vi "CRYTS Step Select.vi"(11 "Tree reference In":refnum<vi>) -> (0 "nData_Out":i32, 2 "sData_Out":string)   [LabVIEW 2013]
uses:
  CRYProject Editor Global.vi
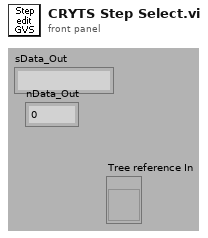
[diagram p1: front panel]
types:
  T1 = typedef "CRYTS.ctl" = cluster{"No.TS":u16, "TS File Path":path, "TS Name":string, "EditStepName":string, "Steps":T2[], "New State":bool, "Change State":bool, "Flattened CurveLib Data":string, "Document Data":string, "EditStepNo":u16, "Operator Start File":string, "Sequence Type":string, "Sequence Language":string}
  T2 = typedef "CRYStep.ctl" = cluster{"No.VI":i32, "Category":string, "StepName":string, "Seq setup flattened":string, "Comment":string, "Steps config.":bool[], "Jump config":i32[], "Start":dbl, "Increment":dbl, "Name":string, "Unit":string, "Y data":u16, "Y prefix":string, "Y dB ref":dbl, "Y unit":string, "Repeat State Array":cluster{"Start":dbl, "Increment":dbl, "Count":i32, "Num":i32}[]}
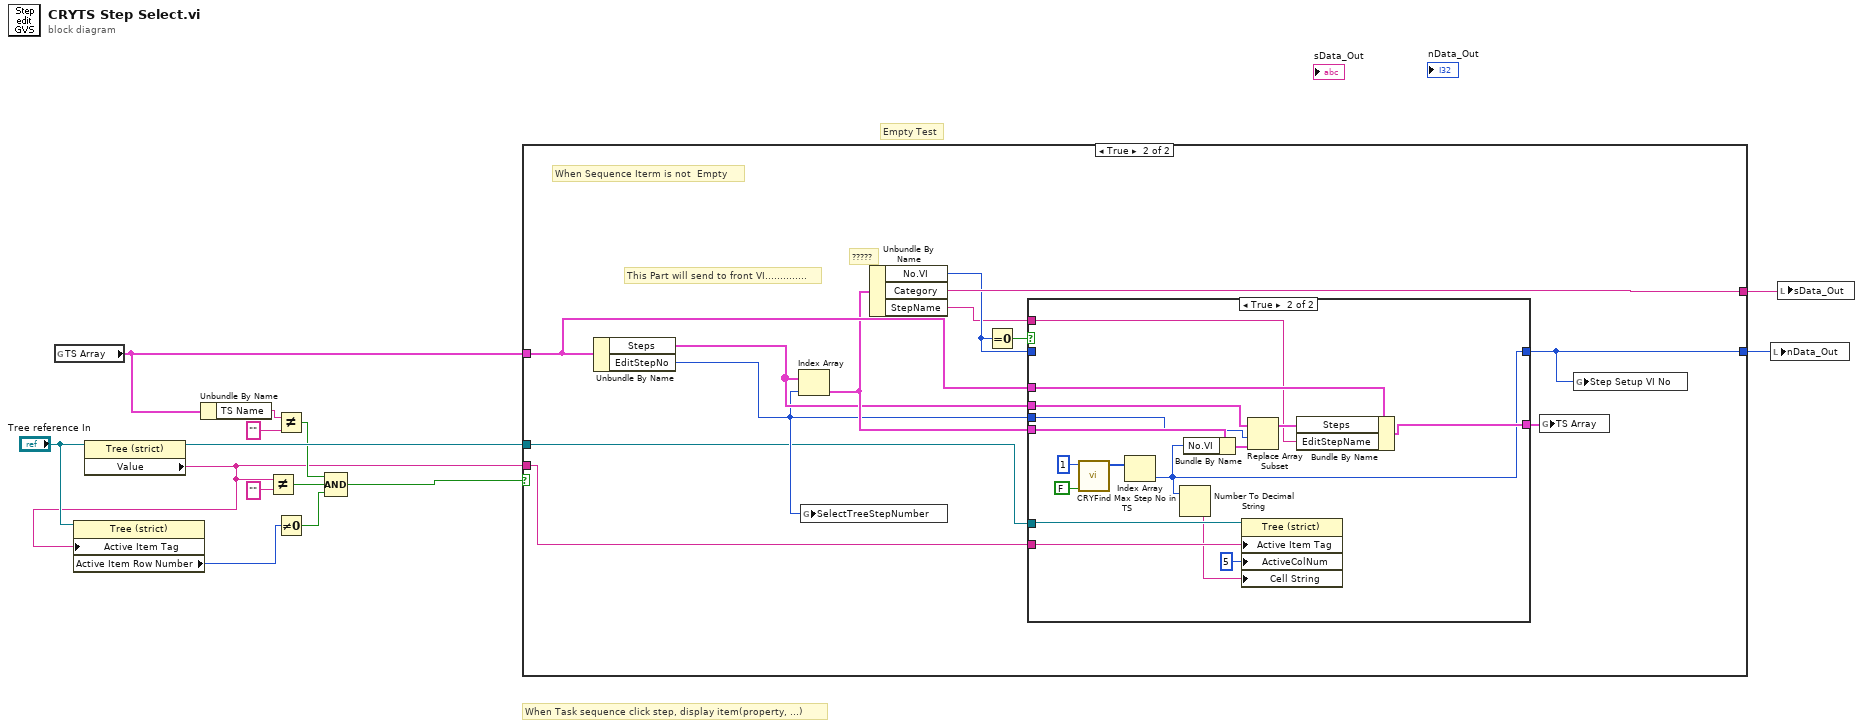
[diagram p0: block diagram]
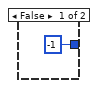
[diagram p2: hidden frame]
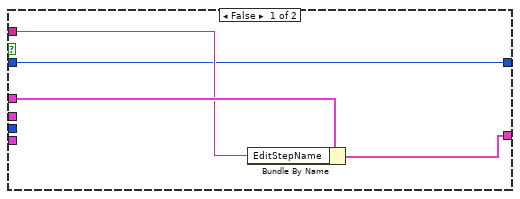
[diagram p3: hidden frame]
diagram:
  # "Empty Test"
  # "When Task sequence click step, display item(property, ...)"
  n1 = global read "CRYProject Editor Global.vi" "TS Array"() -> (w7:T1)
  n2 = property on="Property Node" class="Tree (strict)"(reference="Tree reference In") -> (reference out=w13:refnum<vi>, "Value"=w2:string)  [unwired: 1 in, 1 out]
  n3 = property on="Property Node" class="Tree (strict)"(reference="Tree reference In", "Active Item Tag"=w2) -> ("Active Item Row Number"=w1:i32)  [unwired: 1 in, 2 out]
  n4 = Unbundle By Name(w7) -> ("TS Name"=w12:string)
  n5 = Not Equal?(x=w2, y="") -> (x != y?=w10:bool)
  n6 = Not Equal?(x=w12, y="") -> (x != y?=w9:bool)
  n7 = Not Equal To 0?(x=w1) -> (x != 0?=w4:bool)
  n8 = Compound Arithmetic op=AND(w9, w10, w4) -> (w11:bool)
  n9 = case shown="True" w11 {
    tunnel: w2 -> [_ w16]
    tunnel: w13 -> [_ w17]
    tunnel: [_ w27] -> w6
    tunnel: w7 -> [_ w26]
    tunnel: [-1 ("Max Number") w25] -> w5
    frame False {
    }
    frame True {
      # "This Part will send to front VI.............."
      # "?????"
      # "When Sequence Iterm is not  Empty"
      n10 = Unbundle By Name(w26) -> ("Steps"=w19:T2[], "EditStepNo"=w18:u16)
      n11 = Index Array(array=w19, index=w18) -> (element=w23:T2)
      n12 = global write "CRYProject Editor Global.vi" "SelectTreeStepNumber"(w18) -> ()
      n13 = Unbundle By Name(w23) -> ("No.VI"=w22:i32, "Category"=w27:string, "StepName"=w21:string)
      n14 = Equal To 0?(x=w22) -> (x = 0?=w24:bool)
      n15 = case shown="True" w24 {
        tunnel: [w28 w34] -> w25
        tunnel: w22 -> [w28 _]
        tunnel: w18 -> [_ w37]
        tunnel: w23 -> [_ w47]
        tunnel: w19 -> [_ w45]
        tunnel: w26 -> [w31 w44]
        tunnel: w21 -> [w30 w42]
        tunnel: [w29 w41] -> w20
        tunnel: w17 -> [_ w36]
        tunnel: w16 -> [_ w35]
        frame False {
          n16 = Bundle By Name(cluster=w31, "EditStepName"=w30) -> (w29:T1)
        }
        frame True {
          n17 = call "CRYFind Max Step No in TS.vi"("Inputflg"=FALSE, "Required Count"=1) -> ("Num Array Out"=w39:i32[])  [unwired: 1 in, 8 out]
          n18 = Index Array(array=w39) -> (element=w34:i32)  [unwired: 1 in]
          n19 = Number To Decimal String(number=w34) -> (decimal integer string=w33:string)  [unwired: 1 in]
          n20 = Bundle By Name(cluster=w47, "No.VI"=w34) -> (w46:T2)
          n21 = property class="Tree (strict)"(reference=w36, "Active Item Tag"=w35, "ActiveColNum"=5 ("Active Cell:Active Column Number"), "Cell String"=w33) -> ()  [unwired: 1 in, 2 out]
          n22 = Replace Array Subset(array=w45, new element=w46, index=w37) -> (w43:T2[])
          n23 = Bundle By Name(cluster=w44, "Steps"=w43, "EditStepName"=w42) -> (w41:T1)
        }
      }
      n24 = global write "CRYProject Editor Global.vi" "TS Array"(w20) -> ()
      n25 = global write "CRYProject Editor Global.vi" "Step Setup VI No"(w25) -> ()
    }
  }
  n26 = local write "nData_Out"(w5) -> ()
  n27 = local write "sData_Out"(w6) -> ()
